vi "Angel2Command.vi"(10 "AngelIn":dbl) -> (2 "CommandOut":u8[](array[numeric]) format="%x")   [LabVIEW 2013]
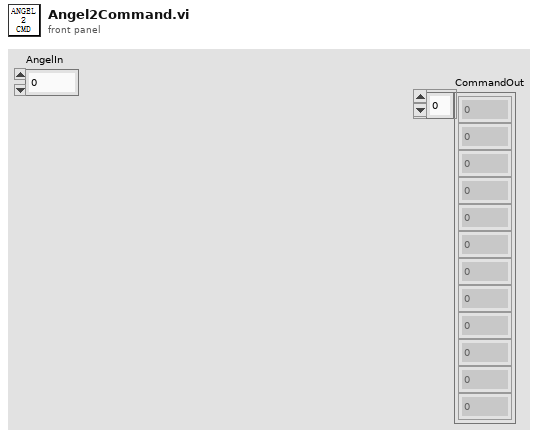
[diagram p1: front panel]
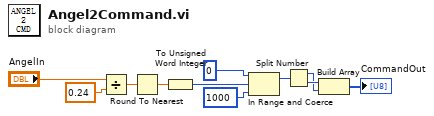
[diagram p0: block diagram]
diagram:
  n1 = Divide(x="AngelIn", y=0.24) -> (x/y=w11:dbl)
  n2 = Round To Nearest(number=w11) -> (nearest integer value=w10:dbl)
  n3 = To Unsigned Word Integer(number=w10) -> (unsigned 16bit integer=w2:u16)
  n4 = In Range and Coerce(upper limit=u16 0, x=w2, lower limit=u16 1000) -> (coerced(x)=w1:u16)  [unwired: 1 out]
  n5 = Split Number(x=w1) -> (hi(x)=w7:u8, lo(x)=w8:u8)
  n6 = Build Array(w8, w7) -> (→"CommandOut":u8[])
